vi "波形图表.vi"() -> ()   [LabVIEW 2018]
panel:
  out "波形图表":dbl(graph)
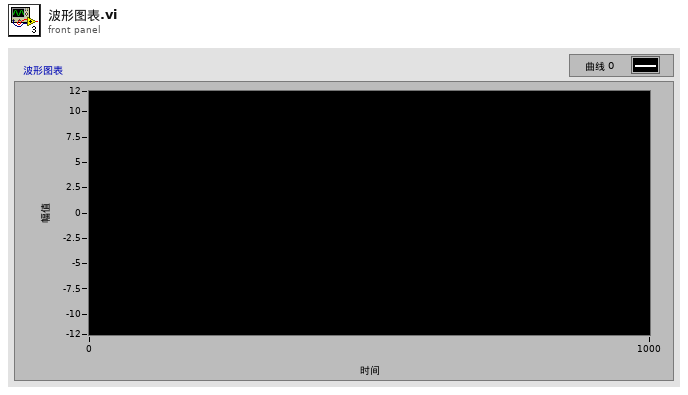
[diagram p1: front panel]
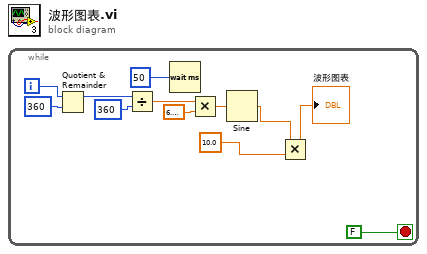
[diagram p0: block diagram]
diagram:
  n1 = while {
    i -> [w12]
    stop <- FALSE stop-if-true
    n2 = Quotient & Remainder(x=w12, y=360) -> (x-y*floor(x/y)=w10:i32)  [unwired: 1 out]
    n3 = Divide(x=w10, y=360) -> (x/y=w8:dbl)
    n4 = Wait (ms)(milliseconds to wait=u32 50 ("毫秒计时值")) -> ()  [unwired: 1 out]
    n5 = Multiply(x=w8, y=6.283185307179586) -> (x*y=w6:dbl)
    n6 = Sine(x=w6) -> (sin(x)=w3:dbl)
    n7 = Multiply(x=w3, y=10.0) -> (x*y=→"波形图表":dbl)
  }
